vi "Sweepback.vi"(4 "Time Between Steps [ms]":dbl, 6 "Step Size [A/V]":dbl, 8 "error in (no error)":errorcluster, 9 "Max reached Current/Voltage [A/V]":dbl, 10 "CC (1)/VC (0)":bool, 11 "VISA resource name":refnum<visa-resource-name>) -> (0 "error out":errorcluster, 3 "VISA resource name out":refnum<visa-resource-name>)   [LabVIEW 2017]
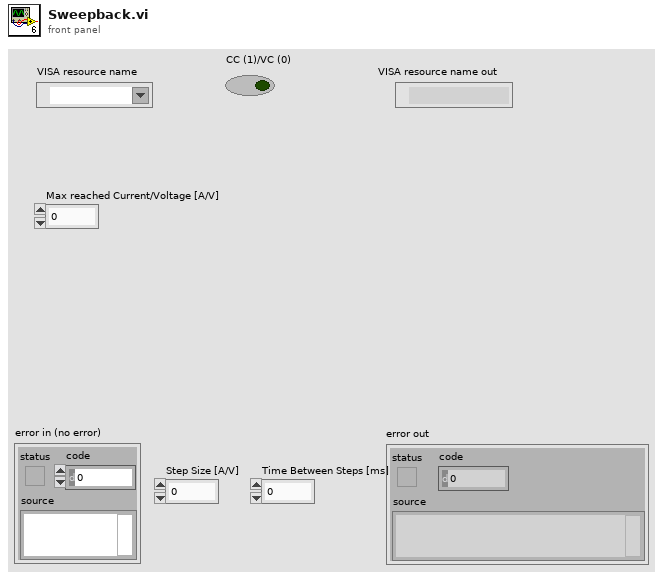
[diagram p1: front panel]
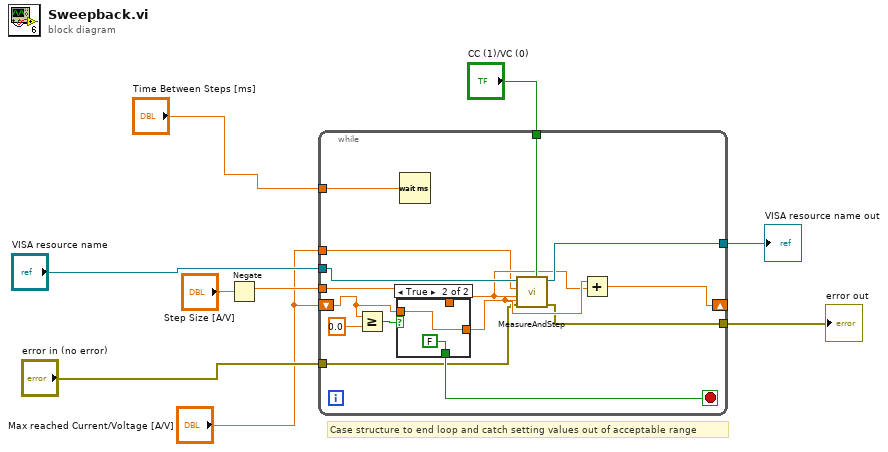
[diagram p0: block diagram]
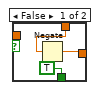
[diagram p2: hidden frame]
diagram:
  # "Case structure to end loop and catch setting values out of acceptable range"
  n1 = Negate(x="Step Size [A/V]") -> (-x=w7:dbl)
  n2 = while {
    tunnel: "CC (1)/VC (0)" -> [w23]
    tunnel: w7 -> [w11]
    shift-right: [w21] -> _
    shift-left: "Max reached Current/Voltage [A/V]" -> [w17]
    tunnel: "Time Between Steps [ms]" -> [w22]
    tunnel: "VISA resource name" -> [w15]
    tunnel: "error in (no error)" -> [w14]
    tunnel: [w13] -> w4
    tunnel: [w12] -> w3
    tunnel: "Max reached Current/Voltage [A/V]" -> [w10]
    stop <- w16 stop-if-true
    n3 = Greater Or Equal?(x=w17, y=0.0) -> (x >= y?=w19:bool)
    n4 = case shown="True" w19 {
      tunnel: [w24 w28] -> w18
      tunnel: w17 -> [_ w28]
      tunnel: [TRUE FALSE] -> w16
      tunnel: w11 -> [w25 _]
      frame False {
        n5 = Negate(x=w25) -> (-x=w24:dbl)
      }
      frame True {
      }
    }
    n6 = Wait (ms)(milliseconds to wait=w22) -> ()  [unwired: 1 out]
    n7 = call "MeasureAndStep.vi"("CC (1)/VC (0)"=w23, "Last Current/Voltage Value (0 A/V)"=w18, "error in (no error)"=w14, "Current/Voltage Step (0 A/V)"=w11, "End Current/Voltage [A/V]"=w10, "VISA resource name"=w15) -> ("error out"=w13:errorcluster, "VISA resource name out"=w12:refnum<visa-resource-name>)  [unwired: 2 in, 2 out]
    n8 = Add(x=w18, y=w11) -> (x+y=w21:dbl)
  }
  "error out" <- w4
  "VISA resource name out" <- w3
